vi "SNMP OID to String.VI"(1 "OID":u8[](array[numeric]) format="%.0x") -> (0 "OID String":string)   [LabVIEW 2017]
doc: "This VI is used to convert the numeric byte array representing an OID to a string representation of the OID. The string representation is the standard dot representation for the OID, e.g. 1.3.4.1.6.1."
panel:
  out "size(s) copy":i32
  out "Bit Array":bool[](array[boolean])
  out "size(s)":i32
  out "Multibyte SubIDFlag":bool
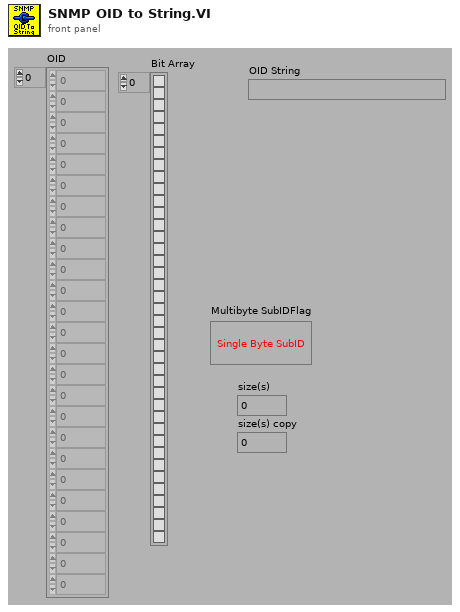
[diagram p1: front panel]
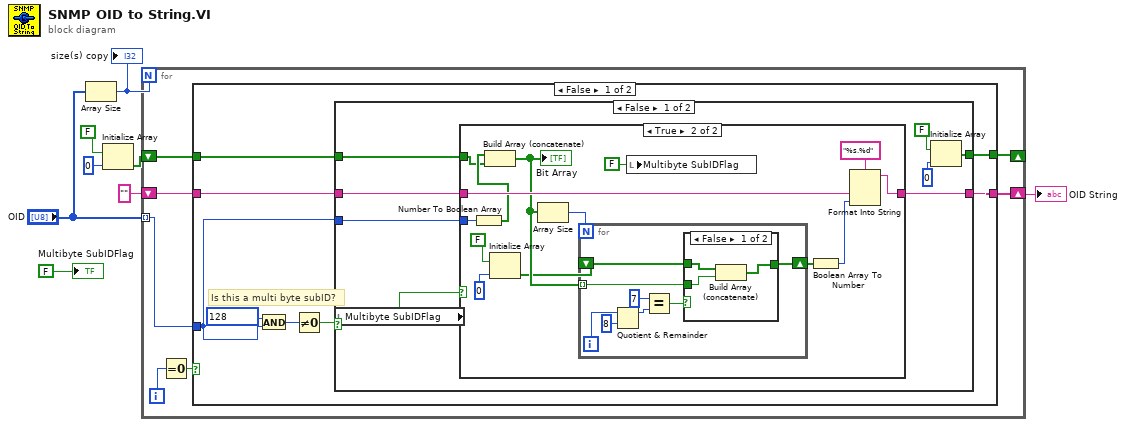
[diagram p0: block diagram]
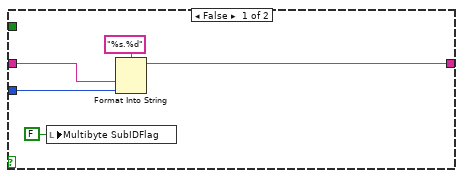
[diagram p2: hidden frame]
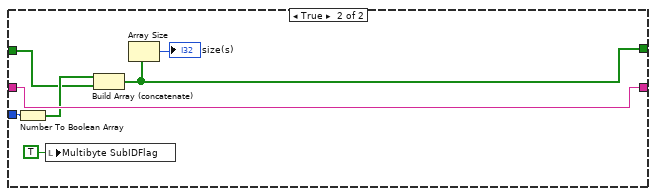
[diagram p4: hidden frame]
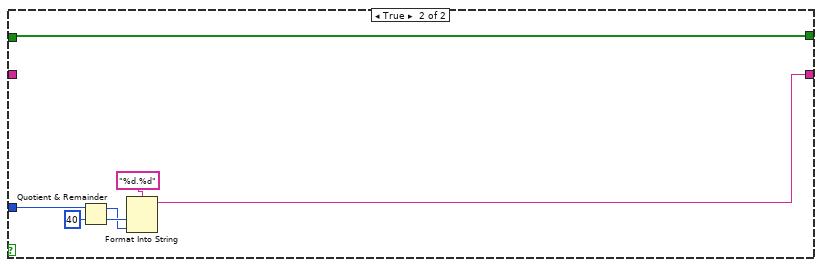
[diagram p5: hidden frame]
diagram:
  n1 = Array Size(array="OID") -> (size(s)=w8:i32)
  "size(s) copy" <- w8
  n2 = Initialize Array(FALSE, 0) -> (w3:bool[])
  n3 = for {
    N: w8 -> [_]
    tunnel: "OID" -> [w15] mode=indexing
    shift-right: [w14] -> _
    shift-left: w3 -> [w11]
    shift-right: [w13] -> w5
    shift-left: "" -> [w12]
    i -> [w10]
    n4 = Equal To 0?(x=w10) -> (x = 0?=w9:bool)
    n5 = case shown="False" w9 {
      tunnel: w15 -> [w20 w76]
      tunnel: [w19 w70] -> w14
      tunnel: [w18 w71] -> w13
      tunnel: w12 -> [w17 _]
      tunnel: w11 -> [w16 w70]
      frame False {
        # "Is this a multi byte subID?"
        n6 = And(x=u8 128, y=w20) -> (x .and. y?=w22:u8)
        n7 = Not Equal To 0?(x=w22) -> (x != 0?=w21:bool)
        n8 = case shown="False" w21 {
          tunnel: w20 -> [w30 w69]
          tunnel: w16 -> [w28 w63]
          tunnel: [w25 w66] -> w19
          tunnel: [w29 w67] -> w18
          tunnel: w17 -> [w24 w67]
          frame False {
            n9 = local read "Multibyte SubIDFlag"() -> (w31:bool)
            n10 = case shown="True" w31 {
              tunnel: w30 -> [w36 w43]
              tunnel: [w35 w44] -> w29
              tunnel: w24 -> [w34 w47]
              tunnel: w28 -> [_ w40]
              frame False {
                n11 = local write "Multibyte SubIDFlag"(FALSE ("Multibyte SubIDFlag")) -> ()
                n12 = Format Into String(format string="%s.%d", w34, w36) -> (resulting string=w35:string)  [unwired: 2 in, 1 out]
              }
              frame True {
                n13 = Number To Boolean Array(number=w43) -> (Boolean array=w41:bool[])
                n14 = Build Array (concatenate)(w41, w40) -> (w42:bool[])
                "Bit Array" <- w42
                n15 = Initialize Array(FALSE, 0) -> (w37:bool[])
                n16 = Array Size(array=w42) -> (size(s)=w49:i32)
                n17 = for {
                  N: w49 -> [_]
                  tunnel: w42 -> [w52] mode=indexing
                  shift-right: [w53] -> w48
                  shift-left: w37 -> [w54]
                  i -> [w58]
                  n18 = Quotient & Remainder(x=w58, y=8) -> (x-y*floor(x/y)=w56:i32)  [unwired: 1 out]
                  n19 = Equal?(x=7, y=w56) -> (x = y?=w51:bool)
                  n20 = case shown="False" w51 {
                    tunnel: w54 -> [w61 w62]
                    tunnel: [w60 w62] -> w53
                    tunnel: w52 -> [w59 _]
                    frame False {
                      n21 = Build Array (concatenate)(w61, w59) -> (w60:bool[])
                    }
                    frame True {
                    }
                  }
                }
                n22 = local write "Multibyte SubIDFlag"(FALSE ("Multibyte SubIDFlag")) -> ()
                n23 = Boolean Array To Number(Boolean array=w48) -> (number=w46:u32)
                n24 = Format Into String(format string="%s.%d", w47, w46) -> (resulting string=w44:string)  [unwired: 2 in, 1 out]
              }
            }
            n25 = Initialize Array(FALSE, 0) -> (w25:bool[])
          }
          frame True {
            n26 = Number To Boolean Array(number=w69) -> (Boolean array=w64:bool[])
            n27 = local write "Multibyte SubIDFlag"(TRUE ("Multibyte SubIDFlag")) -> ()
            n28 = Build Array (concatenate)(w64, w63) -> (w66:bool[])
            n29 = Array Size(array=w66) -> (size(s)=→"size(s)":i32)
          }
        }
      }
      frame True {
        n30 = Quotient & Remainder(x=w76, y=u8 40) -> (x-y*floor(x/y)=w73:u8, floor(x/y)=w74:u8)
        n31 = Format Into String(format string="%d.%d", w74, w73) -> (resulting string=w71:string)  [unwired: 2 in, 1 out]
      }
    }
  }
  "OID String" <- w5
  "Multibyte SubIDFlag" <- FALSE ("Multibyte SubIDFlag")
